vi "Read data.vi"(8 "error in (no error)":errorcluster caption="에러 입력(에러 없음)", 11 "Script Line_i2c 입력":refnum<class "Script Line_i2c.lvclass">) -> (0 "error out":errorcluster caption="에러 출력", 2 "data":u8[](array[numeric]) format="%02x", 3 "Script Line_i2c 출력":refnum<class "Script Line_i2c.lvclass">)   [LabVIEW 2020, in "Script Line_i2c.lvclass"]
uses:
  Script Line_i2c.lvclass
  Script Line_i2c.lvclass/Script Line_i2c.ctl
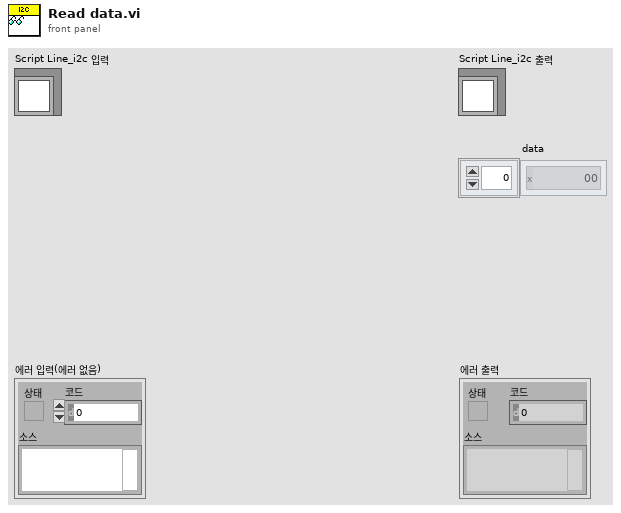
[diagram p1: front panel]
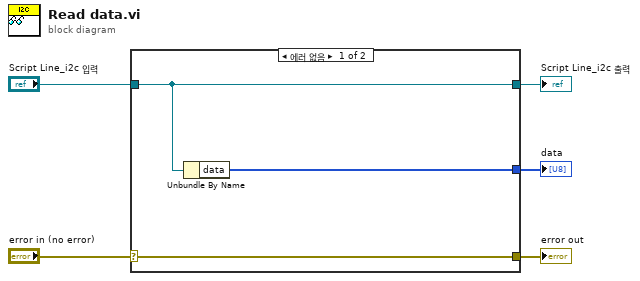
[diagram p0: block diagram]
diagram:
  n1 = case shown="에러 없음" "error in (no error)" {
    selector: "error in (no error)" -> [w8 w9]
    tunnel: [w8 w9] -> w4
    tunnel: [w7 w10] -> w2
    tunnel: "Script Line_i2c 입력" -> [w7 w10]
    tunnel: [w6 _] -> w1
    frame No Error {
      n2 = Unbundle By Name(w7) -> ("data"=w6:u8[])
    }
    frame Error {
    }
  }
  "error out" <- w4
  "Script Line_i2c 출력" <- w2
  "data" <- w1
